vi "Get pin Status.vi"(8 "error in (no error)":errorcluster, 9 "Pin 2":dbl, 10 "Puerto":dbl, 11 "Arduino in":refnum<class "Arduino.lvclass">) -> (0 "error out":errorcluster, 3 "Arduino out":refnum<class "Arduino.lvclass">)   [LabVIEW 2020, in "Arduino.lvclass"]
doc: "Override del papa Get pin status"
uses:
  Arduino.lvclass
  9cba4bcd-0a31-489b-a7c8-93a0bb32cd39.vi
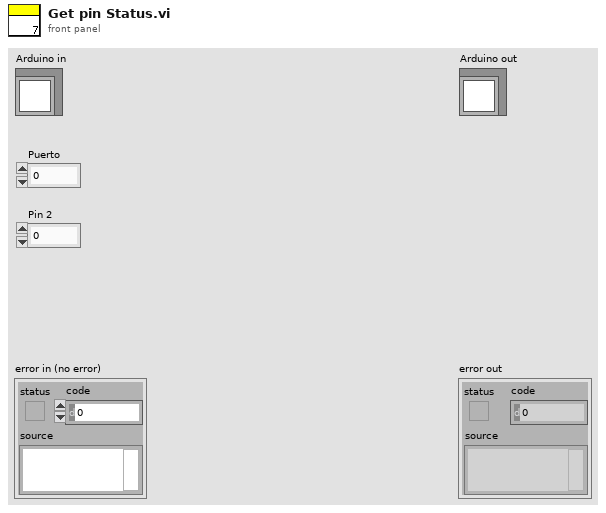
[diagram p1: front panel]
types:
  T1 = typedef "Serial Device.lvclass/serial device brand.ctl" = string
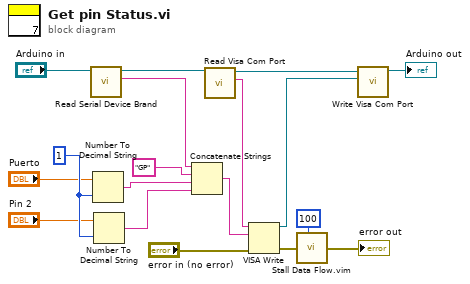
[diagram p0: block diagram]
diagram:
  w14 = i16 1 ("width (-)")
  n1 = call-dynamic "Read Serial Device Brand.vi"("Serial Device in"="Arduino in") -> ("Serial Device Brand"=w5:T1, "Serial Device out"=w17:refnum<class "Arduino.lvclass">)  [unwired: 8 in, 1 out]
  n2 = Number To Decimal String(number="Puerto", width (-)=w14) -> (decimal integer string=w3:string)
  n3 = Number To Decimal String(number="Pin 2", width (-)=w14) -> (decimal integer string=w2:string)
  n4 = Concatenate Strings(w5, "GP" ("string"), w3, w2) -> (w1:string)
  n5 = call-dynamic "Read Visa Com Port.vi"("Serial Device in"=w17) -> ("Visa Com Port"=w8:string, "Serial Device out"=w16:refnum<class "Arduino.lvclass">)  [unwired: 8 in, 1 out]
  n6 = VISA Write(VISA resource name=w8, write buffer=w1, error in (no error)="error in (no error)") -> (VISA resource name out=w7:refnum<visa-resource-name>, error out=w11:errorcluster)  [unwired: 1 out]
  n7 = call "Stall Data Flow.vim"("value in"=w11, "milliseconds to wait"=u32 100) -> ("value out"=→"error out":errorcluster)  [unwired: 1 out]
  n8 = call-dynamic "Write Visa Com Port.vi"("Visa Com Port"=w7, "Serial Device in"=w16) -> ("Serial Device out"=→"Arduino out":refnum<class "Arduino.lvclass">)  [unwired: 8 in, 1 out]
